vi "Write Experiment Description JSON.vi"(8 "error in (no error)":errorcluster, 10 "Experiment Description JSON":string, 11 "Control Experiment":refnum<class "SMO.Control Experiment.lvclass">) -> (0 "error out":errorcluster, 3 "Control Experiment out":refnum<class "SMO.Control Experiment.lvclass">)   [LabVIEW 2019, in "SMO.Control Experiment.lvclass"]
uses:
  SMO.Control Experiment.lvclass
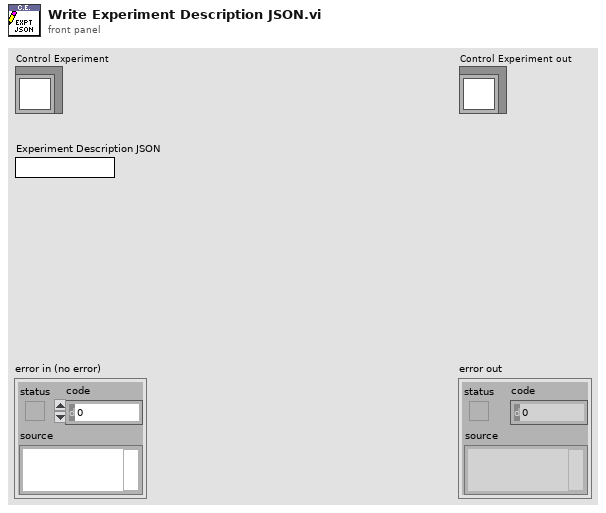
[diagram p1: front panel]
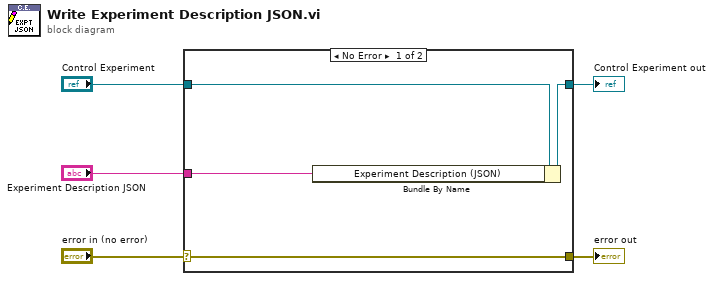
[diagram p0: block diagram]
diagram:
  n1 = case shown="No Error" "error in (no error)" {
    selector: "error in (no error)" -> [w9 w10]
    tunnel: [w9 w10] -> w4
    tunnel: [w6 w11] -> w2
    tunnel: "Control Experiment" -> [w8 w11]
    tunnel: "Experiment Description JSON" -> [w7 _]
    frame No Error {
      n2 = Bundle By Name(cluster=w8, "Experiment Description (JSON)"=w7) -> (w6:refnum<class "SMO.Control Experiment.lvclass">)
    }
    frame Error {
    }
  }
  "error out" <- w4
  "Control Experiment out" <- w2
